vi "Untitled 5 (SubVI).vi"(11 "Numeric":i32) -> (3 "Boolean":bool)   [LabVIEW 2017]
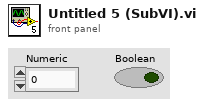
[diagram p1: front panel]
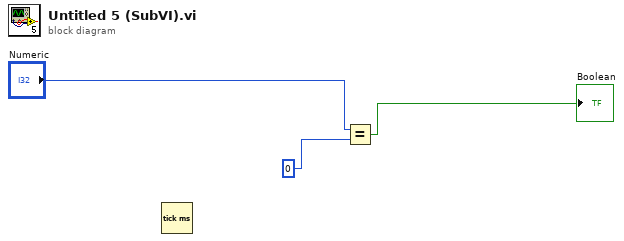
[diagram p0: block diagram]
diagram:
  n1 = Tick Count (ms)() -> ()  [unwired: 1 out]
  n2 = Equal?(x="Numeric", y=0) -> (x = y?=→"Boolean":bool)
